vi "GUI Control Builder Factroy.vi"(8 "error in (no error)":errorcluster, 11 "GUI Control Builder Director in":refnum<class "GUI Control Builder Director.lvclass">) -> (0 "error out":errorcluster, 2 "Control Builder":refnum<class "GUI Control Builder.lvclass">, 3 "GUI Control Builder Director out":refnum<class "GUI Control Builder Director.lvclass">)   [LabVIEW 2015, in "GUI Control Builder Director.lvclass"]
uses:
  GUI Control Builder Director.lvclass
  Control Builders/GUI Control Builder/GUI Control Builder.lvclass
  Panel Control/Panel Data/Type Definition/Panel Control Maker State Variable.ctl
  GUI Control Builder Director.lvclass/GUI Control Builder Director.ctl
  <vilib>/Utility/error.llb/Error Cluster From Error Code.vi
  <vilib>/ErrorRing/Error Ring.xnode
  Panel Control_Ref/Panel Controller.lvclass
panel:
  in  "Cancel?":bool
  in  "Radio Buttons":enum32{"Button", "Parameter", "Graph"}(radio)
  in  "Ok":bool
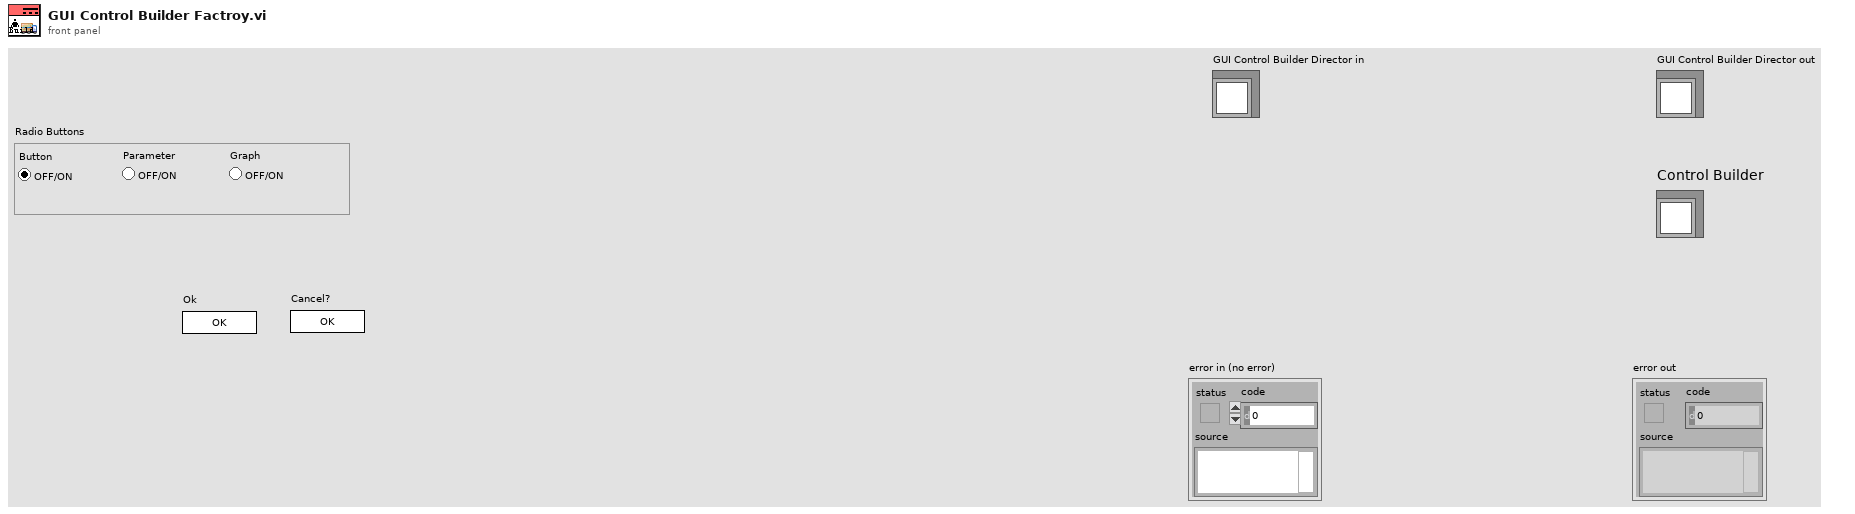
[diagram p1: front panel]
types:
  T1 = typedef "Panel Controller.lvclass/Panel Control Maker State Variable.ctl" = enum16{"Panel On", "Working", "Panel Off", "Ending"}
  T2 = enum32{"Invalid", "Standard", "Closed", "Hidden", "Minimized", "Maximized"}
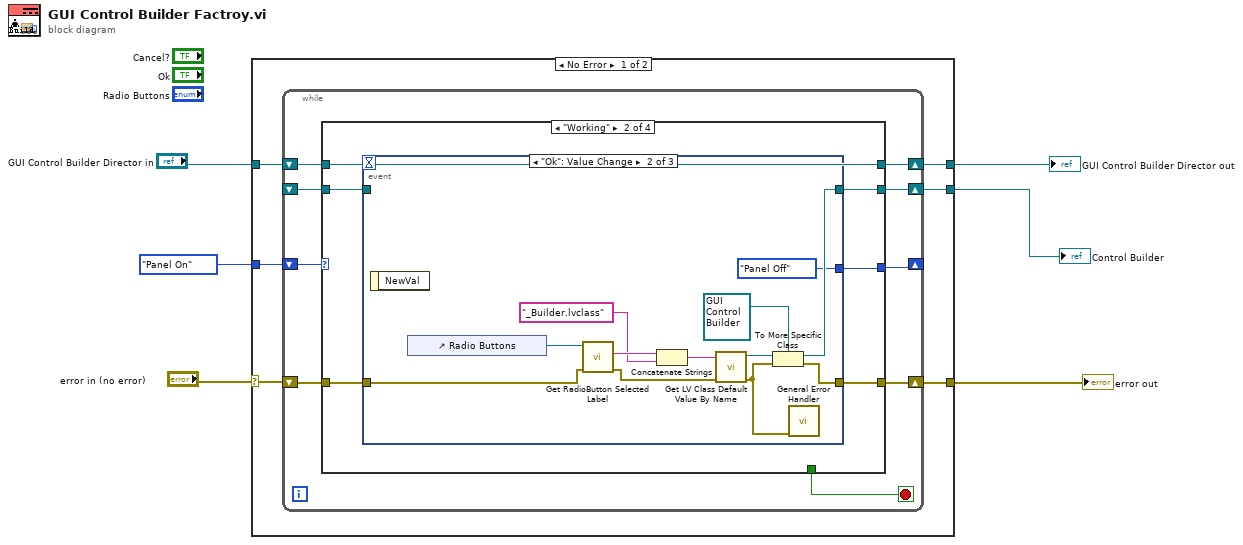
[diagram p0: block diagram]
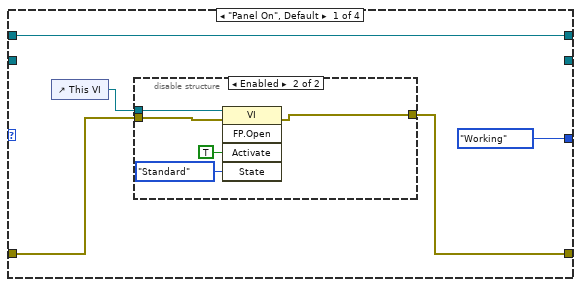
[diagram p2: hidden frame]
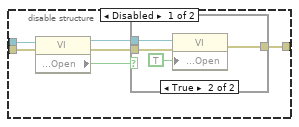
[diagram p3: hidden frame]
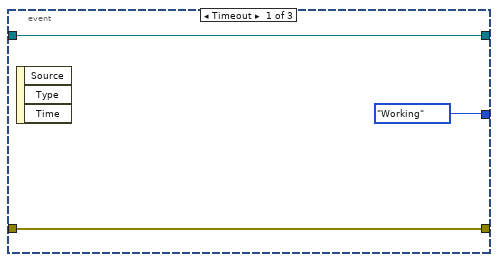
[diagram p5: hidden frame]
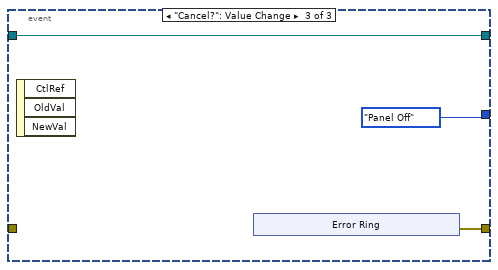
[diagram p6: hidden frame]
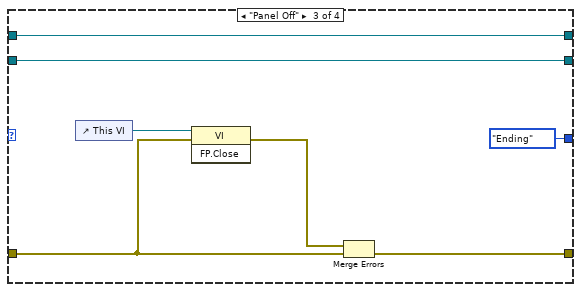
[diagram p7: hidden frame]
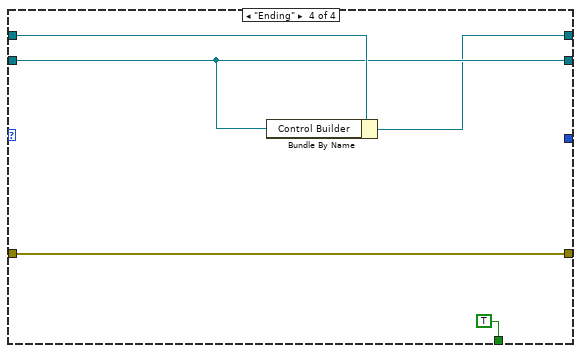
[diagram p8: hidden frame]
diagram:
  n1 = case shown="No Error" "error in (no error)" {
    selector: "error in (no error)" -> [w11 w85]
    tunnel: Panel_Control_Maker_State_Variable."Panel On" -> [w12 _]
    tunnel: [w10 w85] -> w4
    tunnel: [w9 _] -> w1
    tunnel: "GUI Control Builder Director in" -> [w8 w84]
    tunnel: [w7 w84] -> w2
    frame No Error {
      n2 = while {
        shift-right: [w18] -> _
        shift-left: w12 -> [w21]
        shift-right: [w19] -> w10
        shift-left: w11 -> [w20]
        shift-right: [w17] -> w9
        shift-left: _ -> [w16]
        shift-right: [w13] -> w7
        shift-left: w8 -> [w14]
        stop <- w15 stop-if-true
        n3 = case shown="\"Working\"" w21 {
          tunnel: w20 -> [w25 w44 w74 w82]
          tunnel: [w24 w45 w76 w82] -> w19
          tunnel: [Panel_Control_Maker_State_Variable."Working" w46 Panel_Control_Maker_State_Variable."Ending" _] -> w18
          tunnel: [_ w48 w78 w80] -> w17
          tunnel: w16 -> [_ w47 w78 w80]
          tunnel: [_ _ _ TRUE] -> w15
          tunnel: w14 -> [w22 w43 w72 w81]
          tunnel: [w22 w43 w72 w79] -> w13
          frame "Panel On", Default {
            n4 = control-ref of="This VI"() -> (w26:refnum<vi>)
            n5 = disable-structure shown="Enabled" {
              disable-tunnel: w26 -> [w32 w42]
              disable-tunnel: w25 -> [w31 w41]
              disable-tunnel: [w27 w40] -> w24
              frame Disabled {
                n6 = property class="VI"(reference=w32, error in=w31) -> (reference out=w28:refnum<vi>, error out=w29:errorcluster, "Front Panel.Open"=w30:bool)
                n7 = case shown="True" w30 {
                  tunnel: w29 -> [w33 w36]
                  tunnel: w28 -> [_ w37]
                  tunnel: [w33 w34] -> w27
                  frame False {
                  }
                  frame True {
                    n8 = property class="VI"(reference=w37, error in=w36, "Front Panel.Open"=TRUE ("Front Panel Window:Open")) -> (error out=w34:errorcluster)  [unwired: 1 out]
                  }
                }
              }
              frame Enabled {
                n9 = invoke class="VI" method="FP.Open"(reference=w42, error in=w41, "Activate"=TRUE ("Activate?"), "State"=T2."Standard") -> (error out=w40:errorcluster)  [unwired: 1 in, 4 out]
              }
            }
          }
          frame "Working" {
            n10 = event shown="[1] \"Ok\": Value Change" {
              selector: _ -> [_ _ _]
              dyn-events: _ -> [_ _ _]
              timeout: _ -> [_ _ _]
              tunnel: [w49 w58 w66] -> w45
              tunnel: [w50 w57 w65] -> w48
              tunnel: w47 -> [w50 _ w65]
              tunnel: [Panel_Control_Maker_State_Variable."Working" Panel_Control_Maker_State_Variable."Panel Off" Panel_Control_Maker_State_Variable."Panel Off"] -> w46
              tunnel: w44 -> [w49 w55 _]
              event Timeout {
                n11 = event-data() -> ()  [unwired: 1 in, 3 out]
              }
              event "Ok": Value Change {
                n12 = event-data() -> ()  [unwired: 1 in, 1 out]
                n13 = control-ref of="Radio Buttons"() -> (w63:refnum<vi>)
                n14 = call "Get RadioButton Selected Label.vi"("error in (no error)"=w55, "Radio Buttons"=w63) -> ("error out"=w54:errorcluster, "Label.Text"=w62:string)  [unwired: 7 in, 1 out]
                n15 = Concatenate Strings(w62, "_Builder.lvclass" ("string")) -> (w60:string)
                n16 = call <vilib>:"Get LV Class Default Value By Name.vi"("error in (no error)"=w54, "class name"=w60) -> ("error out"=w53:errorcluster, "object"=w59:refnum<class>)  [unwired: 8 in]
                n17 = To More Specific Class(target class=refnum<class "GUI Control Builder.lvclass"> refnum ("Control Builder"), reference=w59, error in=w53) -> (specific class reference=w57:refnum<class "GUI Control Builder.lvclass">, error out=w58:errorcluster)
                n18 = call <vilib>:"General Error Handler.vi"("error in (no error)"=w53) -> ()  [unwired: 10 in, 5 out]
              }
              event "Cancel?": Value Change {
                n19 = event-data() -> ()  [unwired: 1 in, 3 out]
                n20 = xnode "Error Ring"() -> ("error out"=w66:errorcluster)
              }
            }
          }
          frame "Panel Off" {
            n21 = control-ref of="This VI"() -> (w75:refnum<vi>)
            n22 = invoke class="VI" method="FP.Close"(reference=w75, error in=w74) -> (error out=w73:errorcluster)  [unwired: 1 in, 2 out]
            n23 = Merge Errors(w73, w74) -> (w76:errorcluster)
          }
          frame "Ending" {
            n24 = Bundle By Name(cluster=w81, "Control Builder"=w80) -> (w79:refnum<class "GUI Control Builder Director.lvclass">)
          }
        }
      }
    }
    frame Error {
    }
  }
  "GUI Control Builder Director out" <- w2
  "error out" <- w4
  "Control Builder" <- w1
